vi "Parse Sentence_PUBX.vi"(8 "error in (no error)":errorcluster, 11 "PUBX sentence":string) -> (0 "error out":errorcluster, 3 "PUBX_Data":T1)   [LabVIEW 2024]
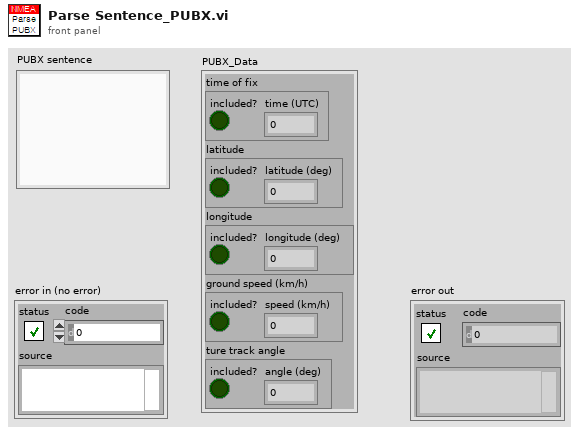
[diagram p1: front panel]
types:
  T1 = cluster{"time of fix":cluster{"included?":bool, "time (UTC)":dbl}, "latitude":cluster{"included?":bool, "latitude (deg)":dbl}, "longitude":cluster{"included?":bool, "longitude (deg)":dbl}, "ground speed (km/h)":cluster{"included?":bool, "speed (km/h)":dbl}, "ture track angle":cluster{"included?":bool, "angle (deg)":dbl}}
  T2 = cluster{"Boolean":bool, "True Track Made Good (Deg)":dbl}
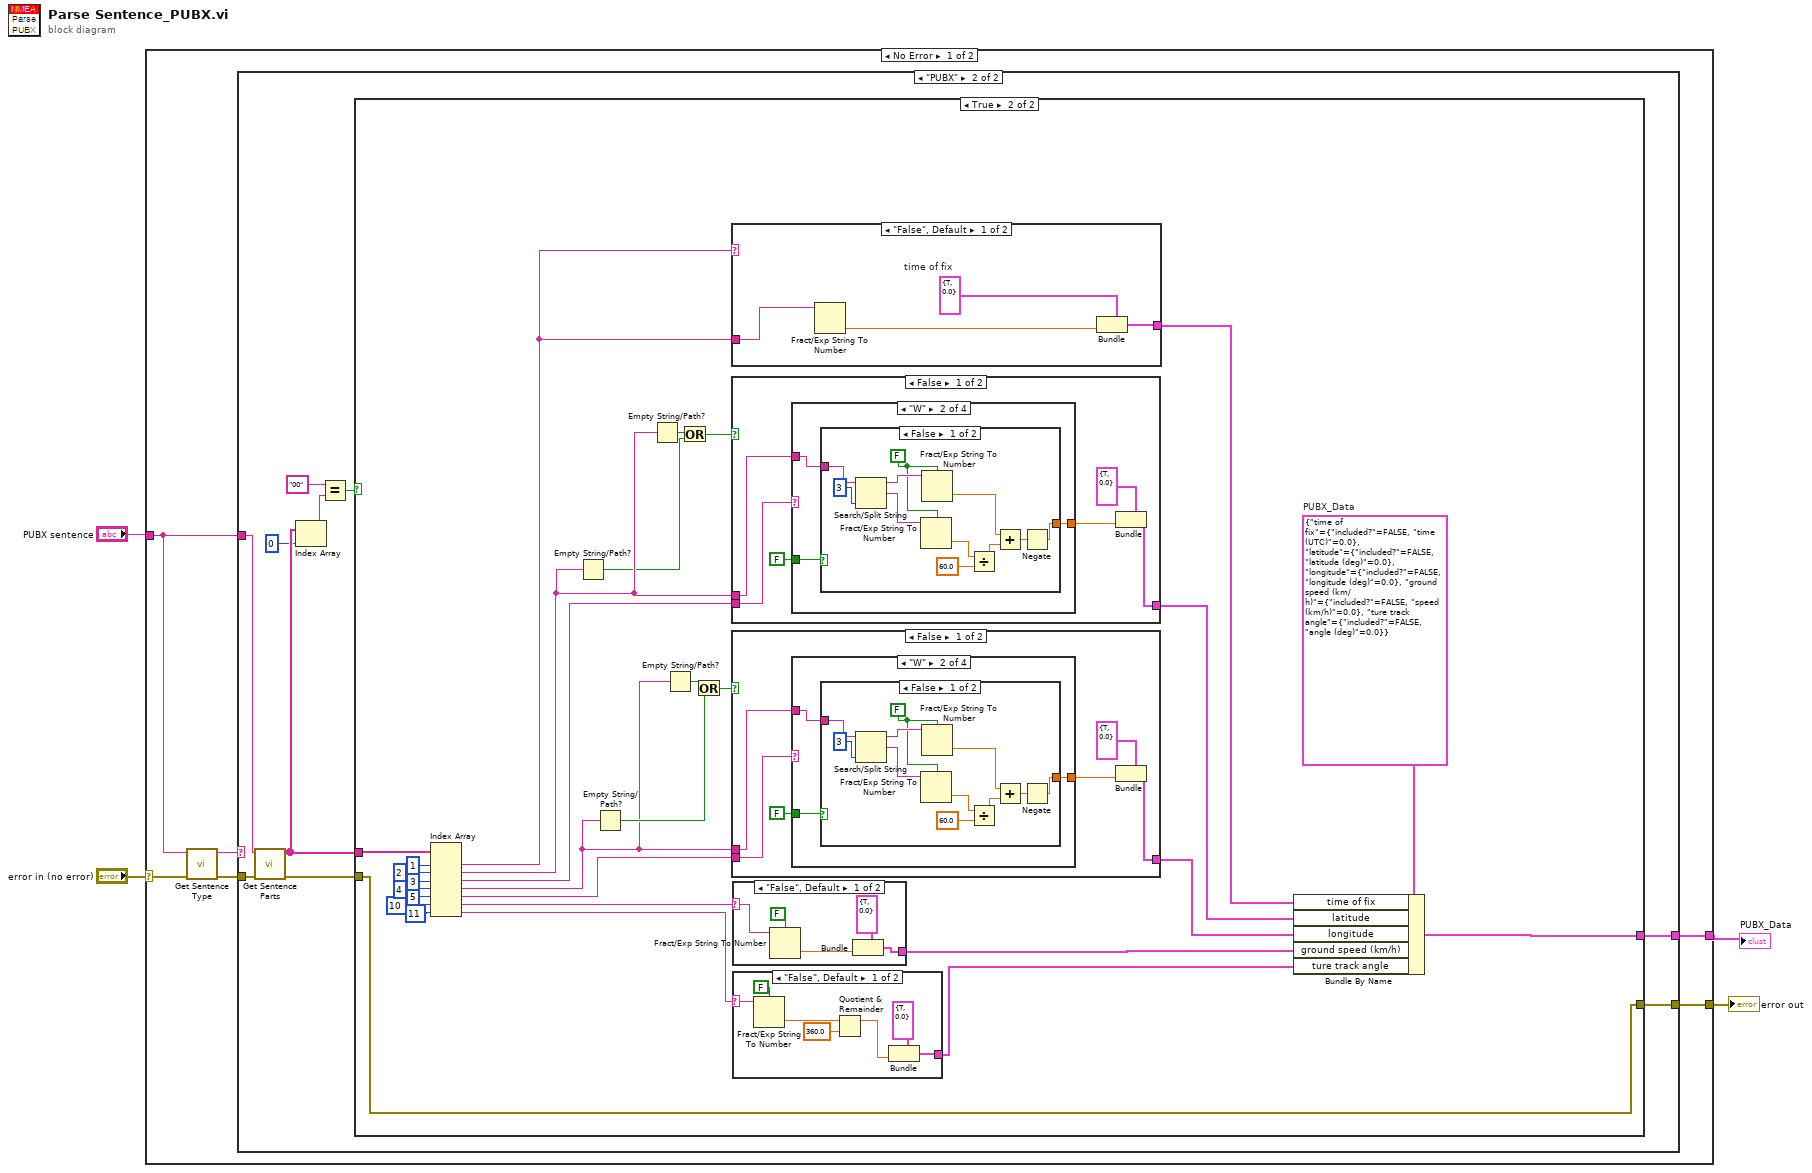
[diagram p0: block diagram]
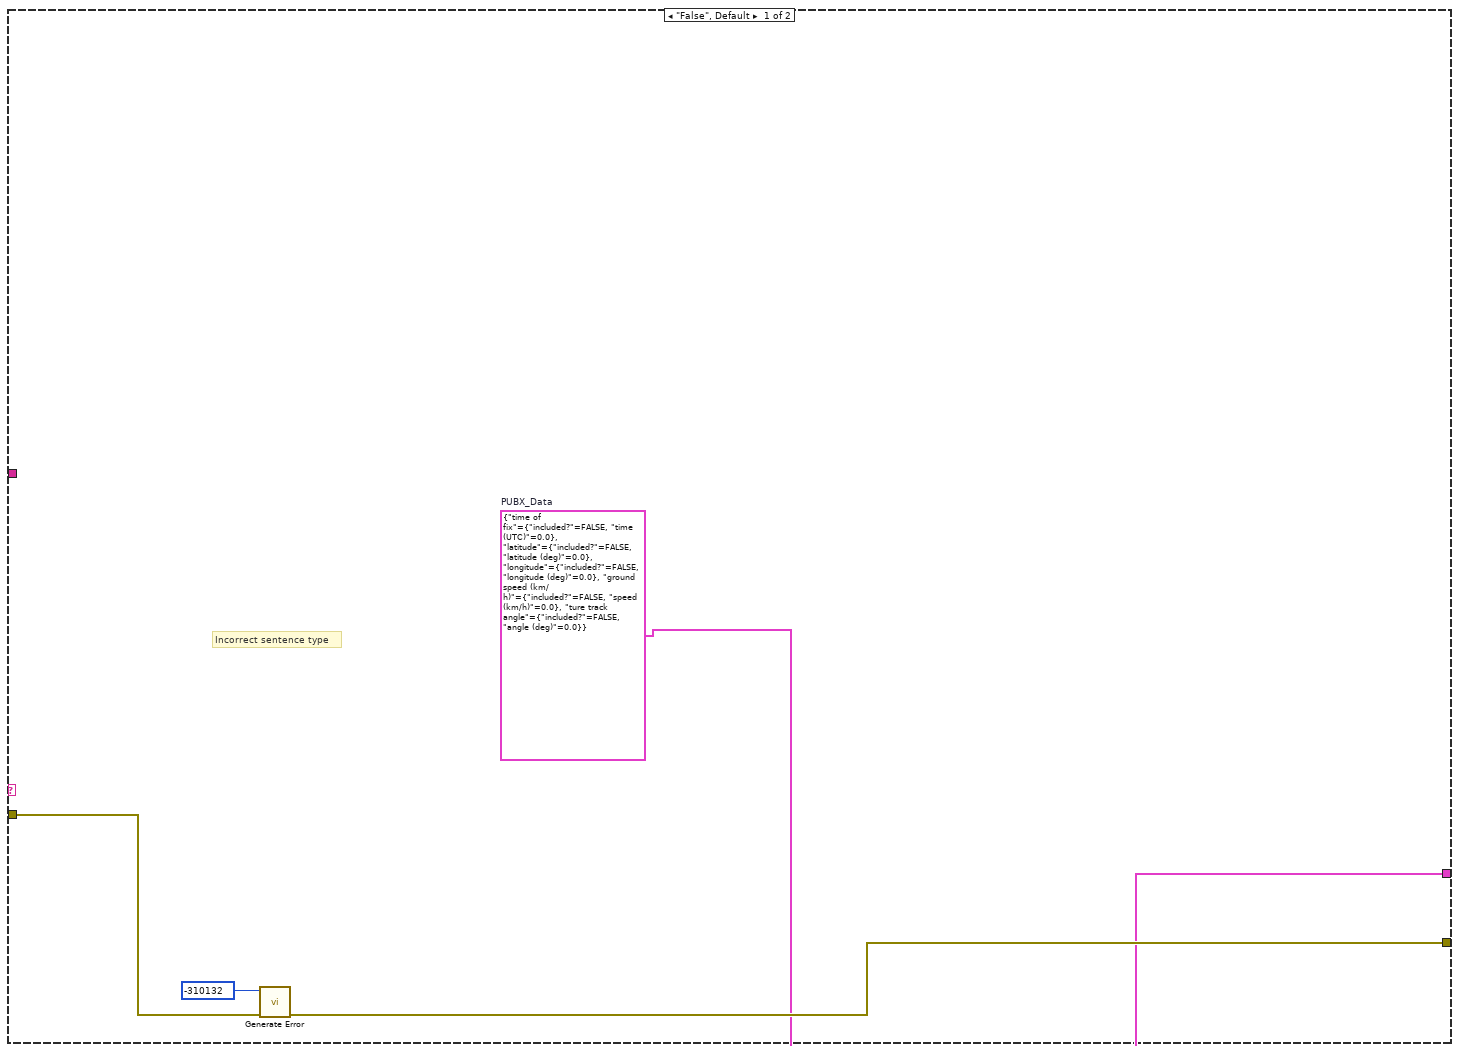
[diagram p2: hidden frame]
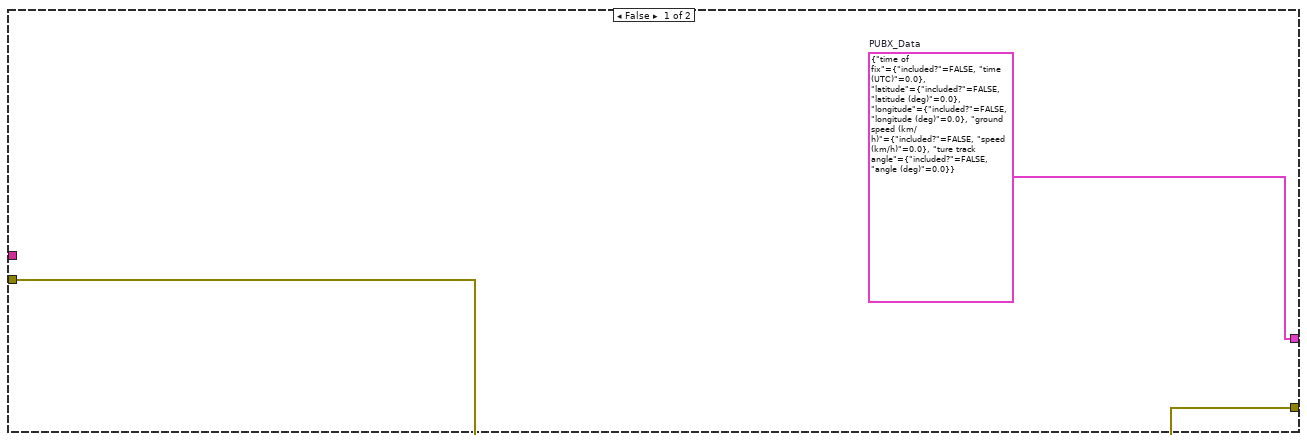
[diagram p3: hidden frame]
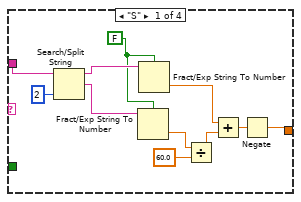
[diagram p4: hidden frame]
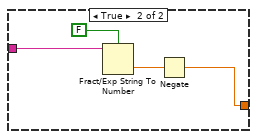
[diagram p5: hidden frame]
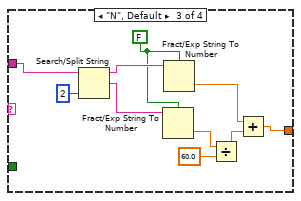
[diagram p6: hidden frame]
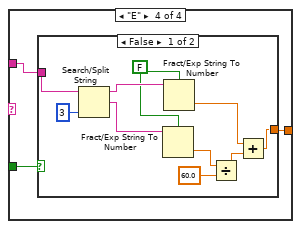
[diagram p7: hidden frame]
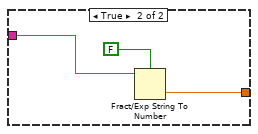
[diagram p8: hidden frame]
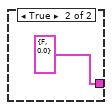
[diagram p9: hidden frame]
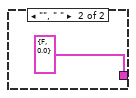
[diagram p10: hidden frame]
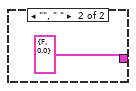
[diagram p11: hidden frame]
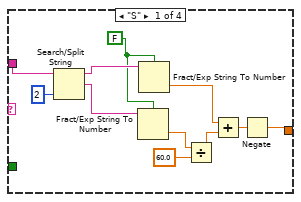
[diagram p12: hidden frame]
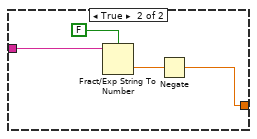
[diagram p13: hidden frame]
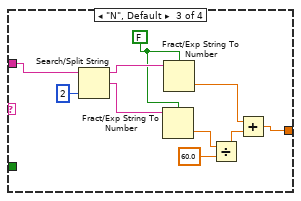
[diagram p14: hidden frame]
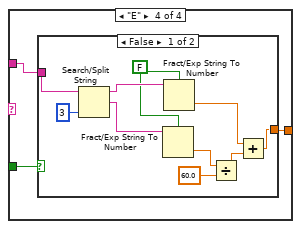
[diagram p15: hidden frame]
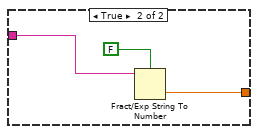
[diagram p16: hidden frame]
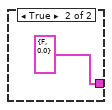
[diagram p17: hidden frame]
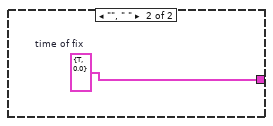
[diagram p18: hidden frame]
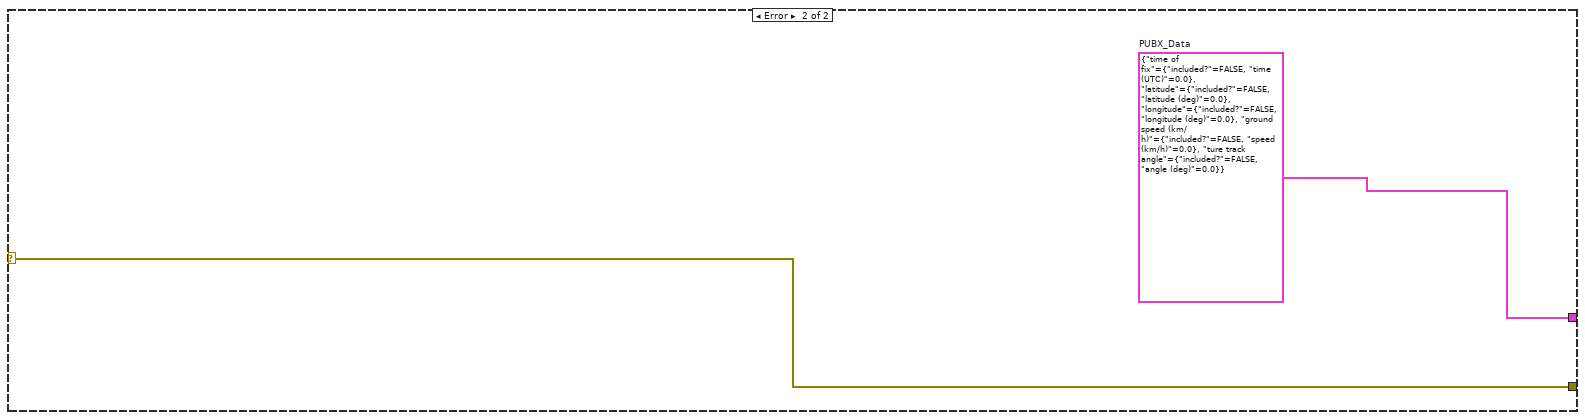
[diagram p19: hidden frame]
diagram:
  n1 = case shown="No Error" "error in (no error)" {
    selector: "error in (no error)" -> [w8 w200]
    tunnel: [w9 w200] -> w2
    tunnel: [w10 w199] -> w1
    tunnel: "PUBX sentence" -> [w6 _]
    frame No Error {
      n2 = call "Get Sentence Type.vi"("error in (no error)"=w8, "sentence"=w6) -> ("error out"=w7:errorcluster, "sentence type"=w5:string)  [unwired: 7 in, 1 out]
      n3 = case shown="\"PUBX\"" w5 {
        tunnel: [w11 w24] -> w10
        tunnel: w6 -> [_ w22]
        tunnel: w7 -> [w13 w23]
        tunnel: [w12 w20] -> w9
        frame "False", Default {
          w11 = T1 {"time of fix"={"included?"=FALSE, "time (UTC)"=0.0}, "latitude"={"included?"=FALSE, "latitude (deg)"=0.0}, "longitude"={"included?"=FALSE, "longitude (deg)"=0.0}, "ground speed (km/h)"={"included?"=FALSE, "speed (km/h)"=0.0}, "ture track angle"={"included?"=FALSE, "angle (deg)"=0.0}}  # PUBX_Data
          # "Incorrect sentence type"
          n4 = call "Generate Error.vi"("error in (no error)"=w13, "code"=-310132) -> ("error out"=w12:errorcluster)  [unwired: 9 in]
        }
        frame "PUBX" {
          n5 = call "Get Sentence Parts.vi"("error in (no error)"=w23, "sentence"=w22) -> ("error out"=w21:errorcluster, "sentence data"=w19:string[])  [unwired: 7 in, 1 out]
          n6 = Index Array(array=w19, index=0) -> (element=w16:string)
          n7 = Equal?(x="00", y=w16) -> (x = y?=w17:bool)
          n8 = case shown="True" w17 {
            tunnel: [w25 w55] -> w24
            tunnel: w19 -> [_ w44]
            tunnel: w21 -> [w26 w37]
            tunnel: [w26 w37] -> w20
            frame False {
              w25 = T1 {"time of fix"={"included?"=FALSE, "time (UTC)"=0.0}, "latitude"={"included?"=FALSE, "latitude (deg)"=0.0}, "longitude"={"included?"=FALSE, "longitude (deg)"=0.0}, "ground speed (km/h)"={"included?"=FALSE, "speed (km/h)"=0.0}, "ture track angle"={"included?"=FALSE, "angle (deg)"=0.0}}  # PUBX_Data
            }
            frame True {
              w43 = T1 {"time of fix"={"included?"=FALSE, "time (UTC)"=0.0}, "latitude"={"included?"=FALSE, "latitude (deg)"=0.0}, "longitude"={"included?"=FALSE, "longitude (deg)"=0.0}, "ground speed (km/h)"={"included?"=FALSE, "speed (km/h)"=0.0}, "ture track angle"={"included?"=FALSE, "angle (deg)"=0.0}}  # PUBX_Data
              n9 = Index Array(array=w44, index #1=1, index #2=2, index #3=3, index #4=4, index #5=5, index #6=10, index #7=11) -> (element #1=w45:string, element #2=w51:string, element #3=w54:string, element #4=w30:string, element #5=w29:string, element #6=w39:string, element #7=w38:string)
              n10 = Empty String/Path?(string/path=w51) -> (empty?=w50:bool)
              n11 = Empty String/Path?(string/path=w30) -> (empty?=w49:bool)
              n12 = Empty String/Path?(string/path=w51) -> (empty?=w52:bool)
              n13 = Empty String/Path?(string/path=w30) -> (empty?=w48:bool)
              n14 = Or(x=w52, y=w50) -> (x .or. y?=w53:bool)
              n15 = Or(x=w48, y=w49) -> (x .or. y?=w27:bool)
              n16 = case shown="\"False\", Default" w45 {
                tunnel: [w197 w198] -> w47
                tunnel: w45 -> [w195 _]
                frame "False", Default {
                  w196 = cluster{"Valid?":bool, "Latitude (Deg)":dbl} {"Valid?"=TRUE, "Latitude (Deg)"=0.0}  # time of fix
                  n17 = Fract/Exp String To Number(string=w195) -> (number=w194:dbl)  [unwired: 4 out]
                  n18 = Bundle(cluster=w196, "Latitude (Deg)"=w194) -> (w197:cluster{"Valid?":bool, "Latitude (Deg)":dbl})  [unwired: 1 out]
                }
                frame "", " " {
                  w198 = cluster{"Valid?":bool, "Latitude (Deg)":dbl} {"Valid?"=TRUE, "Latitude (Deg)"=0.0}  # time of fix
                }
              }
              n19 = case shown="False" w53 {
                tunnel: [w137 cluster{"Valid?":bool, "Latitude (Deg)":dbl} {"Valid?"=FALSE, "Latitude (Deg)"=0.0} ("Latitude")] -> w46
                tunnel: w51 -> [w134 _]
                tunnel: w54 -> [w133 _]
                frame False {
                  n20 = case shown="\"W\"" w133 {
                    tunnel: w134 -> [w141 w151 w176 w179]
                    tunnel: [w139 w150 w168 w178] -> w132
                    tunnel: FALSE -> [_ w149 _ w177]
                    frame "S" {
                      w138 = FALSE ("use system decimal point (T)")
                      n21 = Search/Split String(string=w141, offset (0)=2) -> (substring before match=w147:string, match + rest of string=w146:string)  [unwired: 2 out]
                      n22 = Fract/Exp String To Number(use system decimal point (T)=w138, string=w146) -> (number=w145:dbl)  [unwired: 3 out]
                      n23 = Fract/Exp String To Number(use system decimal point (T)=w138, string=w147) -> (number=w142:dbl)  [unwired: 3 out]
                      n24 = Divide(x=w145, y=60.0) -> (x/y=w143:dbl)
                      n25 = Add(x=w142, y=w143) -> (x+y=w140:dbl)
                      n26 = Negate(x=w140) -> (-x=w139:dbl)
                    }
                    frame "W" {
                      n27 = case shown="False" w149 {
                        tunnel: w151 -> [w155 w166]
                        tunnel: [w153 w164] -> w150
                        frame False {
                          w152 = FALSE ("use system decimal point (T)")
                          n28 = Search/Split String(string=w155, offset (0)=3) -> (substring before match=w161:string, match + rest of string=w160:string)  [unwired: 2 out]
                          n29 = Fract/Exp String To Number(use system decimal point (T)=w152, string=w160) -> (number=w159:dbl)  [unwired: 3 out]
                          n30 = Fract/Exp String To Number(use system decimal point (T)=w152, string=w161) -> (number=w156:dbl)  [unwired: 3 out]
                          n31 = Divide(x=w159, y=60.0) -> (x/y=w157:dbl)
                          n32 = Add(x=w156, y=w157) -> (x+y=w154:dbl)
                          n33 = Negate(x=w154) -> (-x=w153:dbl)
                        }
                        frame True {
                          n34 = Fract/Exp String To Number(use system decimal point (T)=FALSE, string=w166) -> (number=w165:dbl)  [unwired: 3 out]
                          n35 = Negate(x=w165) -> (-x=w164:dbl)
                        }
                      }
                    }
                    frame "N", Default {
                      w167 = FALSE ("use system decimal point (T)")
                      n36 = Search/Split String(string=w176, offset (0)=2) -> (substring before match=w174:string, match + rest of string=w173:string)  [unwired: 2 out]
                      n37 = Fract/Exp String To Number(use system decimal point (T)=w167, string=w173) -> (number=w172:dbl)  [unwired: 3 out]
                      n38 = Fract/Exp String To Number(use system decimal point (T)=w167, string=w174) -> (number=w169:dbl)  [unwired: 3 out]
                      n39 = Divide(x=w172, y=60.0) -> (x/y=w170:dbl)
                      n40 = Add(x=w169, y=w170) -> (x+y=w168:dbl)
                    }
                    frame "E" {
                      n41 = case shown="False" w177 {
                        tunnel: w179 -> [w189 w192]
                        tunnel: [w181 w191] -> w178
                        frame False {
                          w180 = FALSE ("use system decimal point (T)")
                          n42 = Search/Split String(string=w189, offset (0)=3) -> (substring before match=w187:string, match + rest of string=w186:string)  [unwired: 2 out]
                          n43 = Fract/Exp String To Number(use system decimal point (T)=w180, string=w186) -> (number=w185:dbl)  [unwired: 3 out]
                          n44 = Fract/Exp String To Number(use system decimal point (T)=w180, string=w187) -> (number=w182:dbl)  [unwired: 3 out]
                          n45 = Divide(x=w185, y=60.0) -> (x/y=w183:dbl)
                          n46 = Add(x=w182, y=w183) -> (x+y=w181:dbl)
                        }
                        frame True {
                          n47 = Fract/Exp String To Number(use system decimal point (T)=FALSE, string=w192) -> (number=w191:dbl)  [unwired: 3 out]
                        }
                      }
                    }
                  }
                  n48 = Bundle(cluster=cluster{"Valid?":bool, "Latitude (Deg)":dbl} {"Valid?"=TRUE, "Latitude (Deg)"=0.0} ("Latitude"), "Latitude (Deg)"=w132) -> (w137:cluster{"Valid?":bool, "Latitude (Deg)":dbl})  [unwired: 1 out]
                }
                frame True {
                }
              }
              n49 = case shown="False" w27 {
                tunnel: [w61 cluster{"Valid?":bool, "Latitude (Deg)":dbl} {"Valid?"=FALSE, "Latitude (Deg)"=0.0} ("Latitude")] -> w28
                tunnel: w30 -> [w58 _]
                tunnel: w29 -> [w57 _]
                frame False {
                  n50 = case shown="\"W\"" w57 {
                    tunnel: w58 -> [w65 w75 w100 w103]
                    tunnel: [w63 w74 w92 w102] -> w56
                    tunnel: FALSE -> [_ w73 _ w101]
                    frame "S" {
                      w62 = FALSE ("use system decimal point (T)")
                      n51 = Search/Split String(string=w65, offset (0)=2) -> (substring before match=w71:string, match + rest of string=w70:string)  [unwired: 2 out]
                      n52 = Fract/Exp String To Number(use system decimal point (T)=w62, string=w70) -> (number=w69:dbl)  [unwired: 3 out]
                      n53 = Fract/Exp String To Number(use system decimal point (T)=w62, string=w71) -> (number=w66:dbl)  [unwired: 3 out]
                      n54 = Divide(x=w69, y=60.0) -> (x/y=w67:dbl)
                      n55 = Add(x=w66, y=w67) -> (x+y=w64:dbl)
                      n56 = Negate(x=w64) -> (-x=w63:dbl)
                    }
                    frame "W" {
                      n57 = case shown="False" w73 {
                        tunnel: w75 -> [w79 w90]
                        tunnel: [w77 w88] -> w74
                        frame False {
                          w76 = FALSE ("use system decimal point (T)")
                          n58 = Search/Split String(string=w79, offset (0)=3) -> (substring before match=w85:string, match + rest of string=w84:string)  [unwired: 2 out]
                          n59 = Fract/Exp String To Number(use system decimal point (T)=w76, string=w84) -> (number=w83:dbl)  [unwired: 3 out]
                          n60 = Fract/Exp String To Number(use system decimal point (T)=w76, string=w85) -> (number=w80:dbl)  [unwired: 3 out]
                          n61 = Divide(x=w83, y=60.0) -> (x/y=w81:dbl)
                          n62 = Add(x=w80, y=w81) -> (x+y=w78:dbl)
                          n63 = Negate(x=w78) -> (-x=w77:dbl)
                        }
                        frame True {
                          n64 = Fract/Exp String To Number(use system decimal point (T)=FALSE, string=w90) -> (number=w89:dbl)  [unwired: 3 out]
                          n65 = Negate(x=w89) -> (-x=w88:dbl)
                        }
                      }
                    }
                    frame "N", Default {
                      w91 = FALSE ("use system decimal point (T)")
                      n66 = Search/Split String(string=w100, offset (0)=2) -> (substring before match=w98:string, match + rest of string=w97:string)  [unwired: 2 out]
                      n67 = Fract/Exp String To Number(use system decimal point (T)=w91, string=w97) -> (number=w96:dbl)  [unwired: 3 out]
                      n68 = Fract/Exp String To Number(use system decimal point (T)=w91, string=w98) -> (number=w93:dbl)  [unwired: 3 out]
                      n69 = Divide(x=w96, y=60.0) -> (x/y=w94:dbl)
                      n70 = Add(x=w93, y=w94) -> (x+y=w92:dbl)
                    }
                    frame "E" {
                      n71 = case shown="False" w101 {
                        tunnel: w103 -> [w113 w116]
                        tunnel: [w105 w115] -> w102
                        frame False {
                          w104 = FALSE ("use system decimal point (T)")
                          n72 = Search/Split String(string=w113, offset (0)=3) -> (substring before match=w111:string, match + rest of string=w110:string)  [unwired: 2 out]
                          n73 = Fract/Exp String To Number(use system decimal point (T)=w104, string=w110) -> (number=w109:dbl)  [unwired: 3 out]
                          n74 = Fract/Exp String To Number(use system decimal point (T)=w104, string=w111) -> (number=w106:dbl)  [unwired: 3 out]
                          n75 = Divide(x=w109, y=60.0) -> (x/y=w107:dbl)
                          n76 = Add(x=w106, y=w107) -> (x+y=w105:dbl)
                        }
                        frame True {
                          n77 = Fract/Exp String To Number(use system decimal point (T)=FALSE, string=w116) -> (number=w115:dbl)  [unwired: 3 out]
                        }
                      }
                    }
                  }
                  n78 = Bundle(cluster=cluster{"Valid?":bool, "Latitude (Deg)":dbl} {"Valid?"=TRUE, "Latitude (Deg)"=0.0} ("Latitude"), "Latitude (Deg)"=w56) -> (w61:cluster{"Valid?":bool, "Latitude (Deg)":dbl})  [unwired: 1 out]
                }
                frame True {
                }
              }
              n79 = case shown="\"False\", Default" w39 {
                selector: w39 -> [w119 _]
                tunnel: [w120 T2 {"Boolean"=FALSE, "True Track Made Good (Deg)"=0.0} ("True Track Made Good")] -> w42
                frame "False", Default {
                  n80 = Fract/Exp String To Number(use system decimal point (T)=FALSE, string=w119) -> (number=w121:dbl)  [unwired: 3 out]
                  n81 = Bundle(cluster=T2 {"Boolean"=TRUE, "True Track Made Good (Deg)"=0.0} ("True Track Made Good"), "True Track Made Good (Deg)"=w121) -> (w120:T2)  [unwired: 1 out]
                }
                frame "", " " {
                }
              }
              n82 = case shown="\"False\", Default" w38 {
                selector: w38 -> [w128 _]
                tunnel: [w129 T2 {"Boolean"=FALSE, "True Track Made Good (Deg)"=0.0} ("True Track Made Good")] -> w41
                frame "False", Default {
                  n83 = Fract/Exp String To Number(use system decimal point (T)=FALSE, string=w128) -> (number=w127:dbl)  [unwired: 3 out]
                  n84 = Quotient & Remainder(x=w127, y=360.0) -> (x-y*floor(x/y)=w126:dbl)  [unwired: 1 out]
                  n85 = Bundle(cluster=T2 {"Boolean"=TRUE, "True Track Made Good (Deg)"=0.0} ("True Track Made Good"), "True Track Made Good (Deg)"=w126) -> (w129:T2)  [unwired: 1 out]
                }
                frame "", " " {
                }
              }
              n86 = Bundle By Name(cluster=w43, "time of fix"=w47, "latitude"=w46, "longitude"=w28, "ground speed (km/h)"=w42, "ture track angle"=w41) -> (w55:T1)
            }
          }
        }
      }
    }
    frame Error {
      w199 = T1 {"time of fix"={"included?"=FALSE, "time (UTC)"=0.0}, "latitude"={"included?"=FALSE, "latitude (deg)"=0.0}, "longitude"={"included?"=FALSE, "longitude (deg)"=0.0}, "ground speed (km/h)"={"included?"=FALSE, "speed (km/h)"=0.0}, "ture track angle"={"included?"=FALSE, "angle (deg)"=0.0}}  # PUBX_Data
    }
  }
  "error out" <- w2
  "PUBX_Data" <- w1
